vi "Save Metadata.vi"(5 "property value":variant, 7 "name":string, 8 "error in (no error)":errorcluster, 9 "channel name":string, 10 "group name":string, 11 "File in":refnum<class "File.lvclass">) -> (0 "error out":errorcluster, 1 "channel name out":string, 2 "group name out":string, 3 "File out":refnum<class "File.lvclass">)   [LabVIEW 2019, in "File.lvclass"]
uses:
  File.lvclass
  File.lvclass/File.ctl
  Read tdms stream.vi
  Write tdms stream.vi
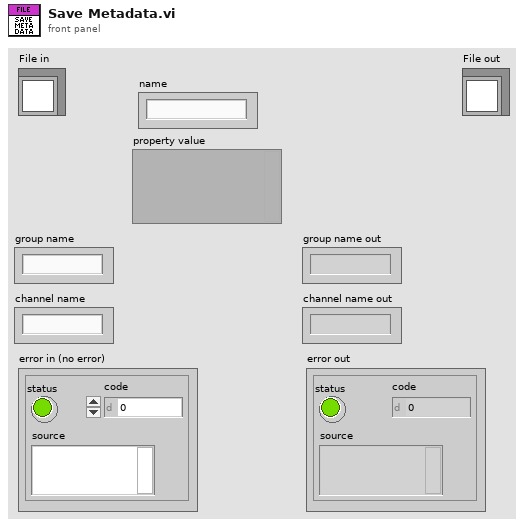
[diagram p1: front panel]
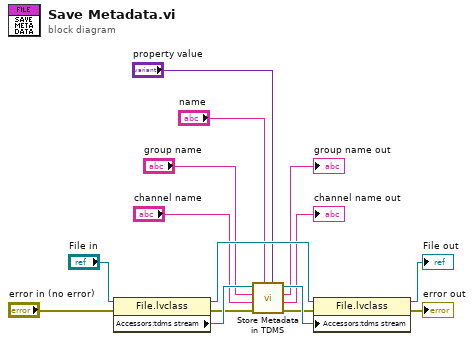
[diagram p0: block diagram]
diagram:
  n1 = property class="File.lvclass"(reference="File in", error in="error in (no error)") -> (reference out=w13:refnum<class "File.lvclass">, error out=w8:errorcluster, "Accessors:tdms stream"=w12:refnum<k34>)
  n2 = call "Store Metadata in TDMS.vi"("Value"="property value", "name"="name", "Error In"=w8, "channel name"="channel name", "group name"="group name", "tdms file"=w12) -> ("Error Out"=w4:errorcluster, "channel name out"=→"channel name out":string, "group name out"=→"group name out":string, "tdms file out"=w5:refnum<k34>)  [unwired: 2 in]
  n3 = property class="File.lvclass"(reference=w13, error in=w4, "Accessors:tdms stream"=w5) -> (reference out=→"File out":refnum<class "File.lvclass">, error out=→"error out":errorcluster)
